vi "Init.vi"() -> (3 "TEMPLATE Msg Output out":refnum<class "TEMPLATE Msg Output.lvclass">)   [LabVIEW 2025, in "_Template.lvlib" / "Templates.lvlib" / "TEMPLATE Msg.lvlib" / "TEMPLATE Msg Output.lvclass"]
uses:
  TEMPLATE Msg Output.lvclass
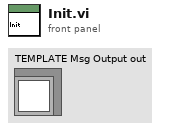
[diagram p1: front panel]
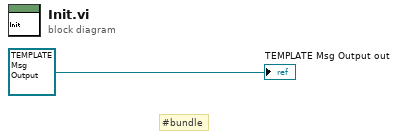
[diagram p0: block diagram]
diagram:
  # "#bundle"
  "TEMPLATE Msg Output out" <- refnum<class "TEMPLATE Msg Output.lvclass"> refnum ("TEMPLATE Msg Output out")
